vi "Read commandName.vi"(8 "error in (no error)":errorcluster, 11 "Disable in":refnum<class "disable.lvclass">) -> (0 "error out":errorcluster, 2 "CommandValue":T1=enum."disable", 3 "Disable out":refnum<class "disable.lvclass">)   [LabVIEW 2016, in "Commands.lvlib" / "disable.lvclass"]
uses:
  disable.lvclass
  Typedefs/CommandValue.ctl
  Typedefs/FiberSpectrographTypedefs.lvlib
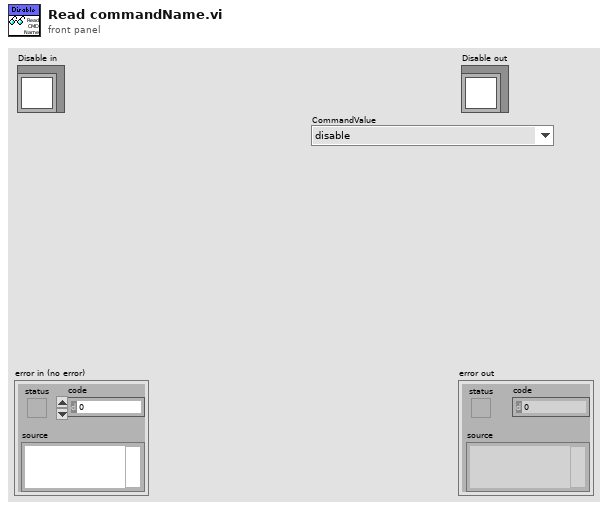
[diagram p1: front panel]
types:
  T1 = typedef "FiberSpectrographTypedefs.lvlib/CommandValue.ctl" = enum16{"clearError", "disable", "enable", "exit", "GoToStandby", "OnHeartbeat", "OnIncomingMessagingError", "OnInterrupt", "start", "captureSpectImage", "setSpectTempSetpoint", "stopImageCapture"}
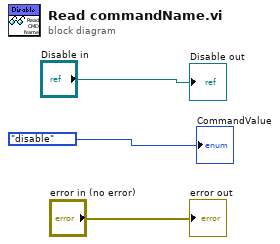
[diagram p0: block diagram]
diagram:
  "error out" <- "error in (no error)"
  "Disable out" <- "Disable in"
  "CommandValue" <- CommandValue."disable" ("CommandValue")
